vi "Minimal Distance to Conjugate Complex Number.vi"(10 "index":i32, 11 "Complex Number Array":cdb[](array[numeric])) -> (2 "min distance to (z)*":dbl, 3 "min distance index":i32)   [LabVIEW 2017, in "NI_AALPro.lvlib"]
uses:
  NI_AALPro.lvlib
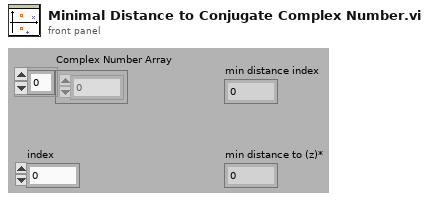
[diagram p1: front panel]
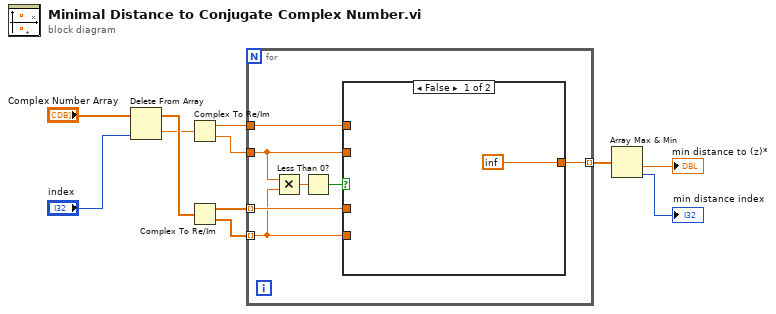
[diagram p0: block diagram]
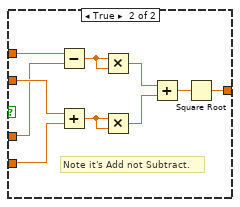
[diagram p2: hidden frame]
diagram:
  n1 = Delete From Array(array="Complex Number Array", index="index") -> (deleted portion=w1:cdb, array with subset deleted=w8:cdb[])  [unwired: 1 in]
  n2 = Complex To Re/Im(x + iy=w1) -> (x=w11:dbl, y=w7:dbl)
  n3 = Complex To Re/Im(x + iy=w8) -> (x=w6:dbl[], y=w5:dbl[])
  n4 = for {
    tunnel: w11 -> [w18]
    tunnel: w7 -> [w16]
    tunnel: w6 -> [w17] mode=indexing
    tunnel: w5 -> [w15] mode=indexing
    tunnel: [w12] -> w4 mode=indexing
    n5 = Multiply(x=w16, y=w15) -> (x*y=w13:dbl)
    n6 = Less Than 0?(x=w13) -> (x < 0?=w14:bool)
    n7 = case shown="False" w14 {
      tunnel: w18 -> [_ w29]
      tunnel: [inf w22] -> w12
      tunnel: w16 -> [_ w23]
      tunnel: w17 -> [_ w21]
      tunnel: w15 -> [_ w20]
      frame False {
      }
      frame True {
        # "Note it's Add not Subtract."
        n8 = Subtract(x=w29, y=w21) -> (x-y=w28:dbl)
        n9 = Add(x=w23, y=w20) -> (x+y=w24:dbl)
        n10 = Multiply(x=w28, y=w28) -> (x*y=w27:dbl)
        n11 = Multiply(x=w24, y=w24) -> (x*y=w26:dbl)
        n12 = Add(x=w27, y=w26) -> (x+y=w25:dbl)
        n13 = Square Root(x=w25) -> (sqrt(x)=w22:dbl)
      }
    }
  }
  n14 = Array Max & Min(array=w4) -> (min value=→"min distance to (z)*":dbl, min index (indices)=→"min distance index":i32)  [unwired: 2 out]
